vi "Agilent VNA Read Sweep Time.vi"(6 "Channel":i8=1 min=1 max=99 step=1, 7 "Agilent VNA":T1, 8 "error in (no error)":errorcluster, 11 "VISA Resource Name":refnum<visa-resource-name>) -> (0 "error out":errorcluster, 2 "Sweep Time, s":dbl=3000.0, 3 "dup VISA Resource Name":refnum<visa-resource-name>)   [LabVIEW 2011]
doc: "This Vi for the HP8753B Network Analyzer is used to set averaging, smoothing, and the IF bandwidth."
uses:
  TypeDefs/Agilent VNA Instrument Info.ctl
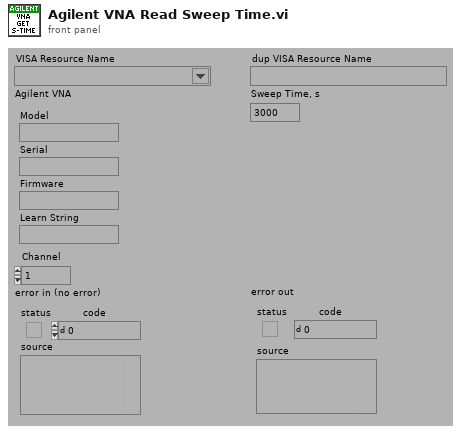
[diagram p1: front panel]
types:
  T1 = typedef "Agilent VNA Instrument Info.ctl" = cluster{"Model":string, "Serial":string, "Firmware":string, "Learn String":string}
  T2 = typedef "Agilent VNA Model.ctl" = enum16{"Not Supported", "8510X", "8719X", "8720X", "8722X", "8753X", "ENA", "PNA", "Field Fox"}
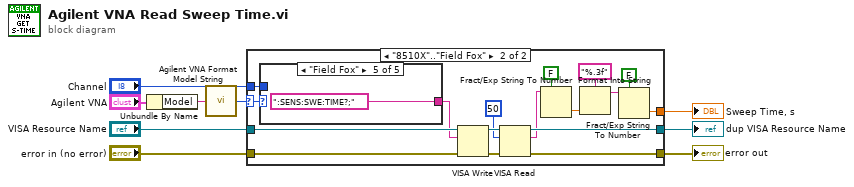
[diagram p0: block diagram]
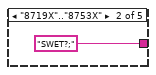
[diagram p4: hidden frame]
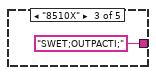
[diagram p5: hidden frame]
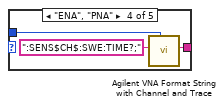
[diagram p6: hidden frame]
diagram:
  n1 = Unbundle By Name("Agilent VNA") -> ("Model"=w2:string)
  n2 = call "Agilent VNA Format Model String.vi"("Model"=w2) -> ("Model"=w1:T2)
  n3 = case shown="\"8510X\"..\"Field Fox\"" w1 {
    selector: w1 -> [_ w12]
    tunnel: "VISA Resource Name" -> [w11 w28]
    tunnel: "error in (no error)" -> [w10 w27]
    tunnel: [w11 w25] -> w7
    tunnel: [w10 w21] -> w6
    tunnel: [_ w15] -> w5
    tunnel: "Channel" -> [_ w13]
    frame "Not Supported" {
    }
    frame "8510X".."Field Fox" {
      n4 = case shown="\"Field Fox\"" w12 {
        tunnel: [_ "SWET?;" "SWET;OUTPACTI;" w32 ":SENS:SWE:TIME?;"] -> w14
        tunnel: w13 -> [_ _ _ w31 _]
        frame "Not Supported" {
        }
        frame "8719X".."8753X" {
        }
        frame "8510X" {
        }
        frame "ENA", "PNA" {
          n5 = call "Agilent VNA Format String with Channel and Trace.vi"("Channel"=w31, "String"=":SENS$CH$:SWE:TIME?;") -> ("String Out"=w32:string)  [unwired: 1 in, 6 out]
        }
        frame "Field Fox" {
        }
      }
      n6 = VISA Write(VISA resource name=w28, write buffer=w14, error in (no error)=w27) -> (VISA resource name out=w26:refnum<visa-resource-name>, error out=w22:errorcluster)  [unwired: 1 out]
      n7 = VISA Read(VISA resource name=w26, byte count=u32 50, error in (no error)=w22) -> (VISA resource name out=w25:refnum<visa-resource-name>, read buffer=w17:string, error out=w21:errorcluster)  [unwired: 1 out]
      n8 = Fract/Exp String To Number(use system decimal point (T)=FALSE, string=w17) -> (number=w20:dbl)  [unwired: 3 out]
      n9 = Format Into String(format string="%.3f", w20) -> (resulting string=w19:string)  [unwired: 2 in, 1 out]
      n10 = Fract/Exp String To Number(use system decimal point (T)=FALSE, string=w19) -> (number=w15:dbl)  [unwired: 3 out]
    }
  }
  "error out" <- w6
  "dup VISA Resource Name" <- w7
  "Sweep Time, s" <- w5
